vi "FTW-File-ValidateFilepath.vi"(1 "Filepath":path) -> (0 "Valid?":bool)   [LabVIEW 2012]
panel:
  # "Inputs"
  # "Outputs"
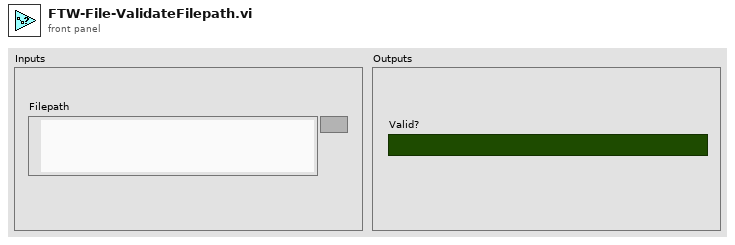
[diagram p1: front panel]
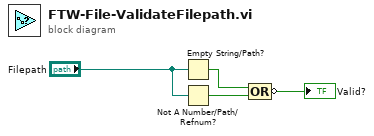
[diagram p0: block diagram]
diagram:
  n1 = Empty String/Path?(string/path="Filepath") -> (empty?=w3:bool)
  n2 = Not A Number/Path/Refnum?(number/path/refnum="Filepath") -> (NaN/Path/Refnum?=w2:bool)
  n3 = Compound Arithmetic op=OR(w3, w2) -> (invert →"Valid?":bool)
